vi "programa8_generacion de temperaturas.vi"() -> ()   [LabVIEW 2013]
panel:
  out "Menor":dbl
  out "Mayor":dbl
  out "Promedio":dbl
  out "Temperatura":i32(slide) scale=0.0..60.0
  # "Generar 10 temperaturas y al final presentar la temperatura mayor, menor y la temperatura promedio"
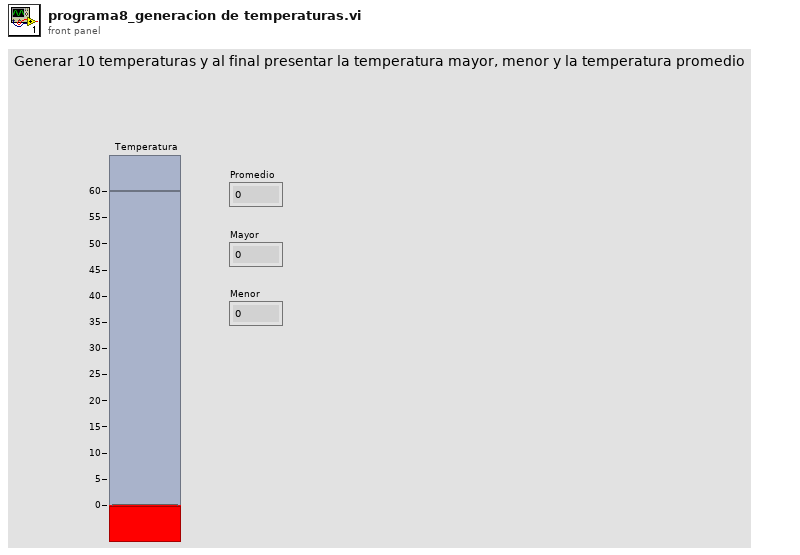
[diagram p1: front panel]
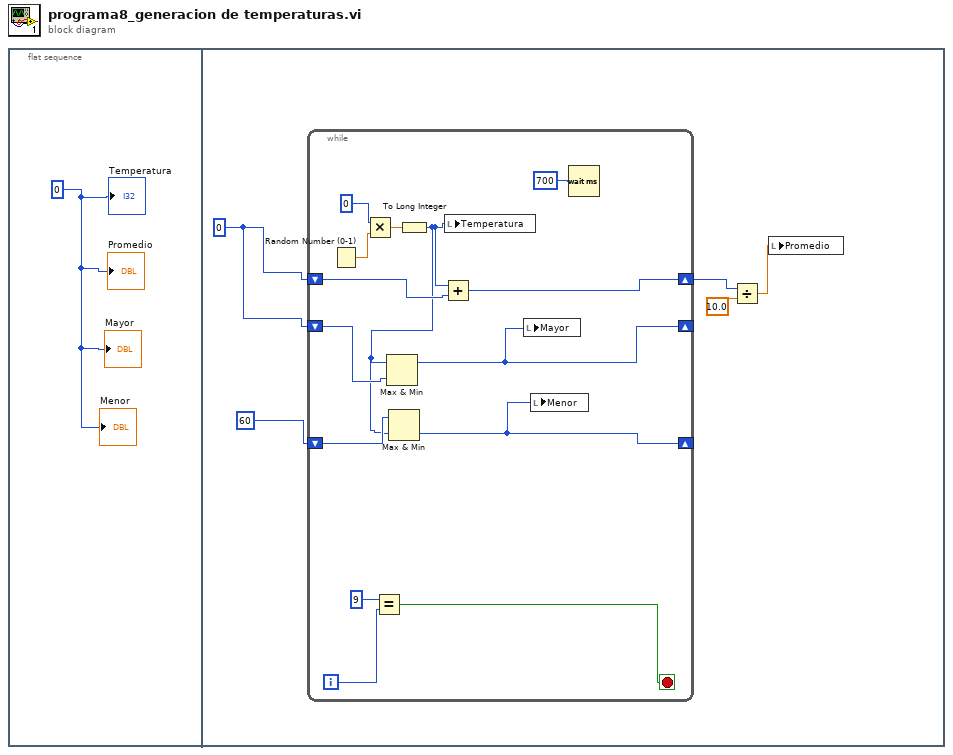
[diagram p0: block diagram]
diagram:
  n1 = flat-sequence {
    frame #0 {
      w1 = 0 ("Temperatura")
      "Temperatura" <- w1
      "Promedio" <- w1
      "Mayor" <- w1
      "Menor" <- w1
    }
    frame #1 {
      w2 = 0
      n2 = while {
        shift-right: [w16] -> w5
        shift-left: w2 -> [w17]
        shift-right: [w12] -> _
        shift-left: w2 -> [w14]
        shift-right: [w11] -> _
        shift-left: 60 -> [w13]
        i -> [w9]
        stop <- w7 stop-if-true
        n3 = Random Number (0-1)() -> (number: 0 to 1=w18:dbl)
        n4 = Multiply(x=0, y=w18) -> (x*y=w20:dbl)
        n5 = Equal?(x=9, y=w9) -> (x = y?=w7:bool)
        n6 = To Long Integer(number=w20) -> (32bit integer=w10:i32)
        n7 = Max & Min(x=w10, y=w14) -> (max(x,y)=w12:i32)  [unwired: 1 out]
        n8 = Max & Min(x=w13, y=w10) -> (min(x,y)=w11:i32)  [unwired: 1 out]
        n9 = Add(x=w10, y=w17) -> (x+y=w16:i32)
        n10 = local write "Temperatura"(w10) -> ()
        n11 = local write "Mayor"(w12) -> ()
        n12 = local write "Menor"(w11) -> ()
        n13 = Wait (ms)(milliseconds to wait=700) -> ()  [unwired: 1 out]
      }
      n14 = Divide(x=w5, y=10.0) -> (x/y=w4:dbl)
      n15 = local write "Promedio"(w4) -> ()
    }
  }
